vi "dist_eqn.vi"(8 "error in":errorcluster, 9 "b2_s":dbl[](array[numeric])=[1.0, 3.0], 10 "b1_s":dbl[](array[numeric])=[1.0, 3.0]) -> (0 "error out":errorcluster, 2 "r":dbl)   [LabVIEW 2020]
panel:
  # "Calculate the r distance value between\ntwo points (bodies)"
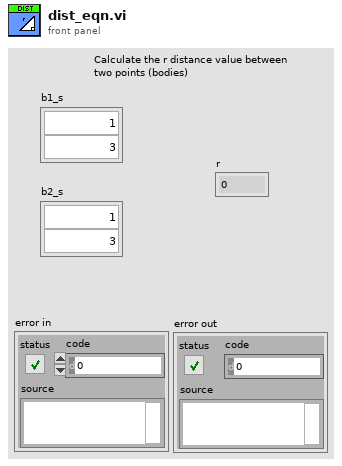
[diagram p1: front panel]
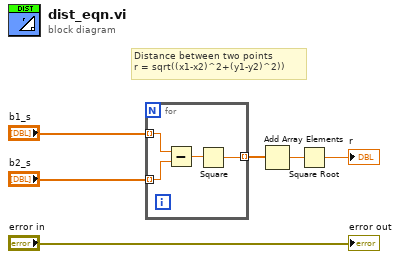
[diagram p0: block diagram]
diagram:
  # "Distance between two points\nr = sqrt((x1-x2)^2+(y1-y2)^2))"
  n1 = for {
    tunnel: "b1_s" -> [w10] mode=indexing
    tunnel: "b2_s" -> [w9] mode=indexing
    tunnel: [w7] -> w4 mode=indexing
    n2 = Subtract(x=w10, y=w9) -> (x-y=w8:dbl)
    n3 = Square(x=w8) -> (x^2=w7:dbl)
  }
  n4 = Add Array Elements(numeric array=w4) -> (sum=w3:dbl)
  n5 = Square Root(x=w3) -> (sqrt(x)=→"r":dbl)
  "error out" <- "error in"
